vi "Handle Command.vi"(8 "error in (no error)":errorcluster, 9 "Data":variant, 10 "Command":string, 11 "Instrument.Oxford1820 in":refnum<class "Instrument.Oxford1820.lvclass">) -> (0 "error out":errorcluster, 1 "Processed Data":variant, 2 "Command":string, 3 "Instrument.Oxford1820 out":refnum<class "Instrument.Oxford1820.lvclass">)   [LabVIEW 2016, in "Instrument.Oxford1820.lvclass"]
uses:
  Instrument.Oxford1820.lvclass
  Typedefs/Instrument.Oxford1820.Commands-enum.ctl
  <instrlib>/Mercury iXX/Public/Libraries/Magnet/Controls/PSU Actions.ctl
  Typedefs/Targets.ctl
  Typedefs/PrivateEvents--Instrument.Oxford1820.SequenceSetMagnetField.ctl
  Typedefs/Instrument.Oxford1820.setMagnet-cluster.ctl
  <userlib>/LevyLab/Levylab Instruments/Instrument Types/Cryostat/Instrument.Cryostat.lvclass
  <instrlib>/Mercury iXX/Public/Libraries/Magnet.lvlib
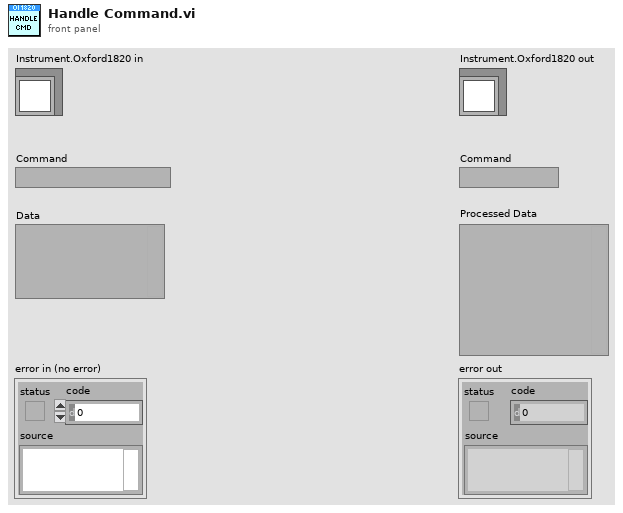
[diagram p1: front panel]
types:
  T1 = typedef "Instrument.Oxford1820.lvclass/Instrument.Oxford1820.Commands-enum.ctl" = enum16{"setAction", "setTarget", "setSwitchHeat", "setLambda", "setFillMode", "setNeedleValve", "setMagnetField", "getStatus", "getTarget", "getSwitchHeat", "getPSUField", "newcommand", "getMagnetField"}
  T2 = typedef "Mercury iXX.lvlib/Magnet.lvlib/PSU Actions.ctl" = string
  T3 = typedef "Instrument.Oxford1820.lvclass/Targets.ctl" = cluster{"Field (T)":dbl, "Field Rate (T/min)":dbl}
  T4 = typedef "Instrument.Oxford1820.lvclass/Instrument.Oxford1820.setMagnet-cluster.ctl" = cluster{"Target":T3, "persistent mode":bool}
  T5 = typedef "Instrument.Oxford1820.lvclass/PrivateEvents--Instrument.Oxford1820.SequenceSetMagnetField.ctl" = cluster{"setMagnet":T4}
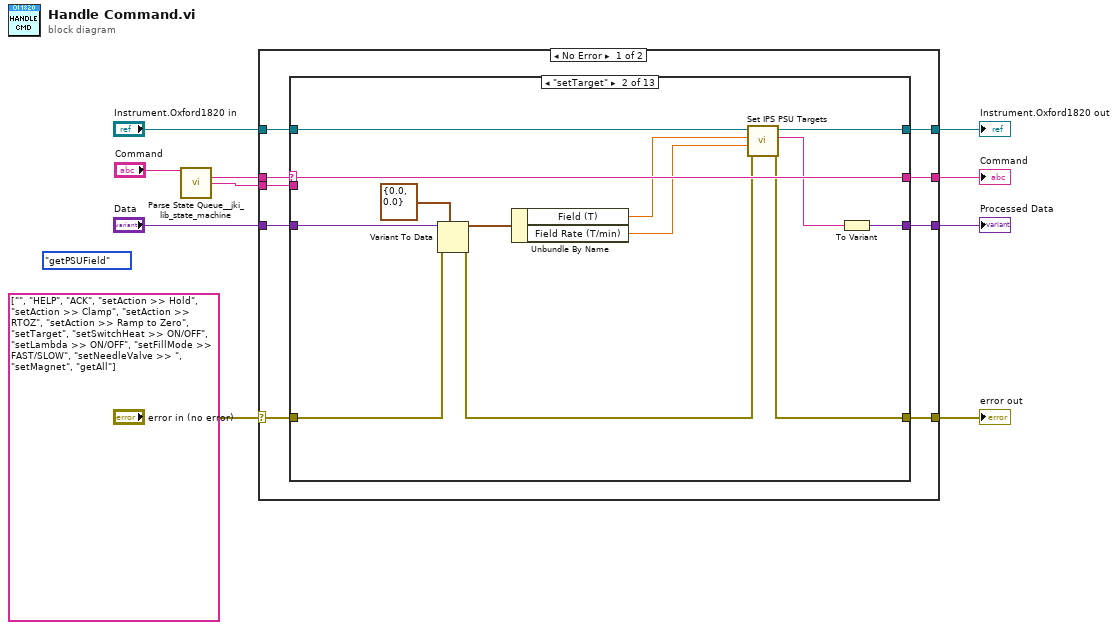
[diagram p0: block diagram]
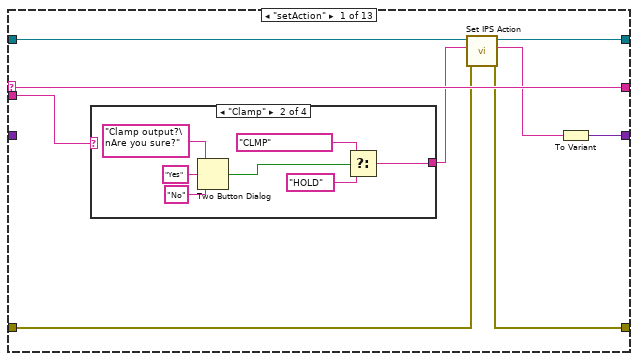
[diagram p2: hidden frame]
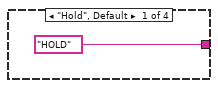
[diagram p3: hidden frame]
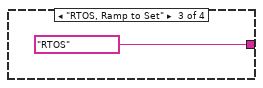
[diagram p4: hidden frame]
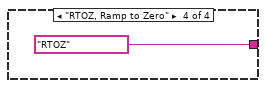
[diagram p5: hidden frame]
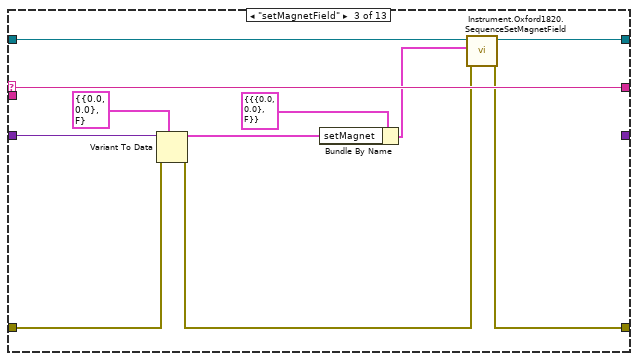
[diagram p6: hidden frame]
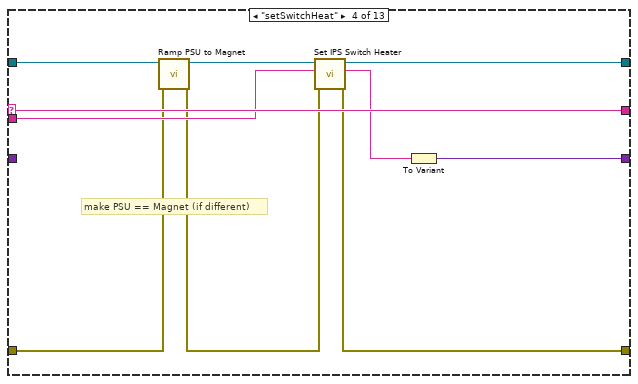
[diagram p7: hidden frame]
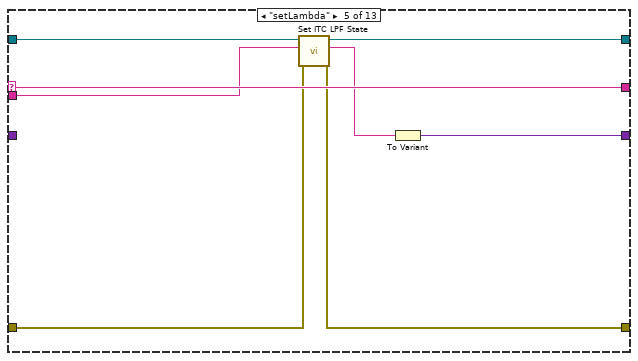
[diagram p8: hidden frame]
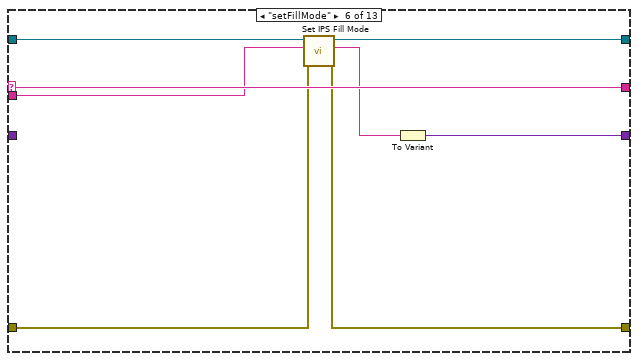
[diagram p9: hidden frame]
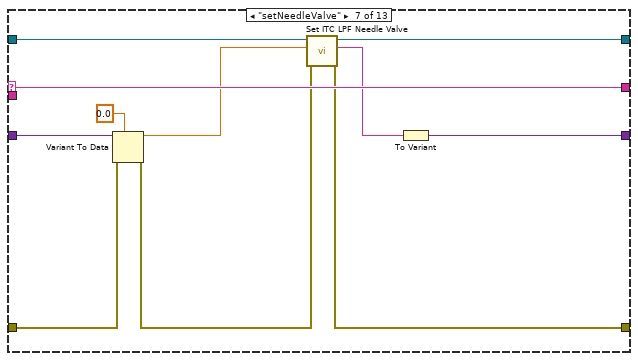
[diagram p10: hidden frame]
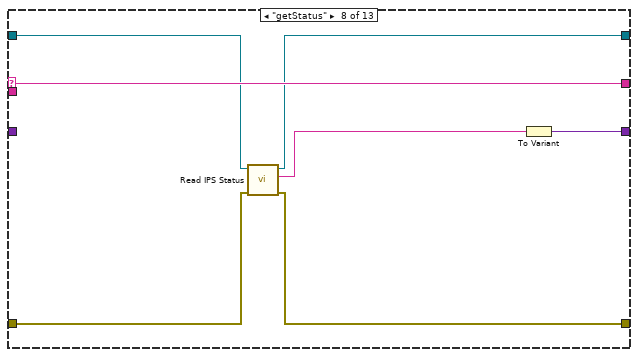
[diagram p11: hidden frame]
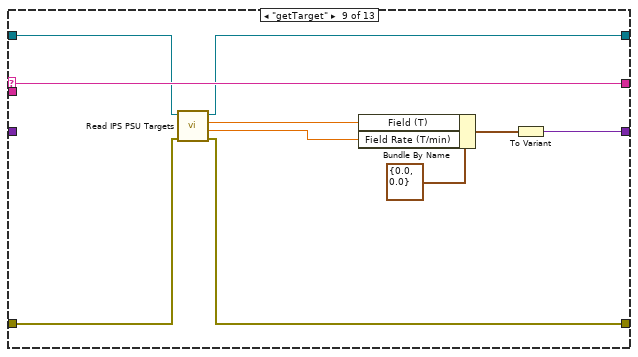
[diagram p12: hidden frame]
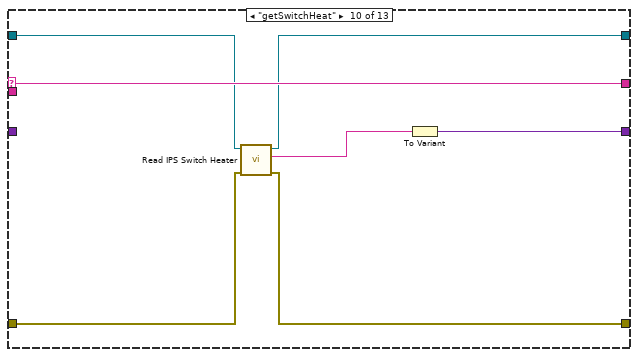
[diagram p13: hidden frame]
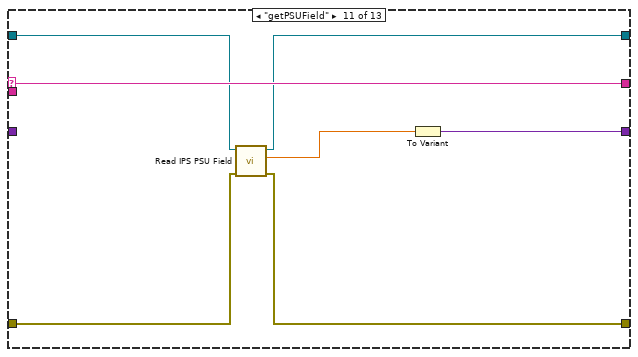
[diagram p14: hidden frame]
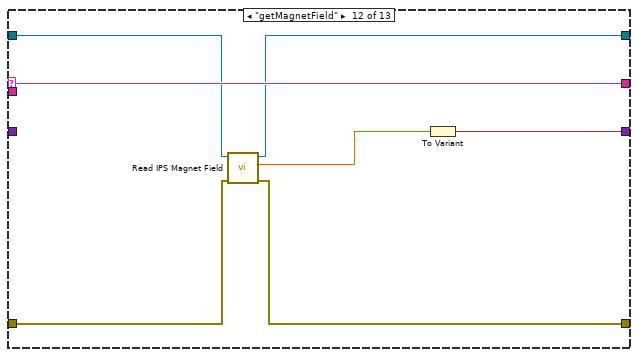
[diagram p15: hidden frame]
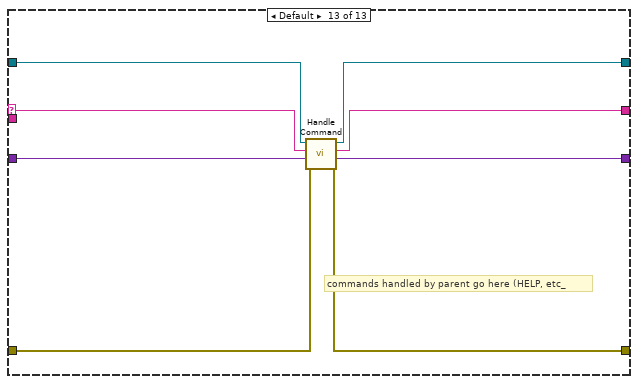
[diagram p16: hidden frame]
diagram:
  (unwired) Instrument.Oxford1820.Commands-enum."getPSUField" ("Commands")
  (unwired) string[] ["", "HELP", "ACK", "setAction >> Hold", "setAction >> Clamp", "setAction >> RTOZ", "setAction >> Ramp to Zero", "setTarget", "setSwitchHeat >> ON/OFF", "setLambda >> ON/OFF", "setFillMode >> FAST/SLOW", "setNeedleValve >> ", "setMagnet", "getAll"] ("Commands")
  n1 = call <vilib>:"Parse State Queue__jki_lib_state_machine.vi"("State Queue"="Command") -> ("Current State"=w2:string, "Arguments"=w1:string)  [unwired: 12 in, 1 out]
  n2 = case shown="No Error" "error in (no error)" {
    selector: "error in (no error)" -> [w14 w146]
    tunnel: [w13 w146] -> w10
    tunnel: [w19 _] -> w9
    tunnel: [w18 _] -> w8
    tunnel: [w17 w147] -> w7
    tunnel: "Data" -> [w16 _]
    tunnel: w2 -> [w11 _]
    tunnel: "Instrument.Oxford1820 in" -> [w15 w147]
    tunnel: w1 -> [w12 _]
    frame No Error {
      n3 = case shown="\"setTarget\"" w11 {
        selector: w11 -> [w28 w51 w62 w72 w80 w88 w99 w106 w116 w123 w130 w137 w138]
        tunnel: [w20 w46 _ w68 w75 w83 w94 w105 w115 w122 w129 w136 w145] -> w19
        tunnel: [w28 w51 w62 w72 w80 w88 w99 w106 w116 w123 w130 w137 w144] -> w18
        tunnel: [w25 w49 w60 w71 w78 w86 w97 w100 w108 w120 w127 w135 w143] -> w17
        tunnel: w16 -> [_ w45 w58 _ _ _ w92 _ _ _ _ _ w142]
        tunnel: w15 -> [w26 w50 w61 w66 w79 w87 w98 w101 w107 w121 w128 w131 w141]
        tunnel: w14 -> [w24 w40 w57 w64 w74 w82 w90 w104 w110 w119 w126 w133 w140]
        tunnel: [w23 w48 w59 w70 w77 w85 w96 w103 w109 w118 w125 w132 w139] -> w13
        tunnel: w12 -> [w27 _ _ w67 w73 w81 _ _ _ _ _ _ _]
        frame "setAction" {
          n4 = case shown="\"Clamp\"" w27 {
            tunnel: [T2 "HOLD" ("PSU Act Stat") w35 T2 "RTOS" ("PSU Act Stat") T2 "RTOZ" ("PSU Act Stat")] -> w22
            frame "Hold", Default {
            }
            frame "Clamp" {
              n5 = Two Button Dialog(message="Clamp output?\nAre you sure?", 1:"No" ("F button name (\"Cancel\")"), 2:"Yes" ("T button name (\"OK\")")) -> (T button?=w34:bool)
              n6 = Select(t=T2 "CLMP" ("PSU Act Stat"), s=w34, f=T2 "HOLD" ("PSU Act Stat")) -> (s? t:f=w35:T2)
            }
            frame "RTOS, Ramp to Set" {
            }
            frame "RTOZ, Ramp to Zero" {
            }
          }
          n7 = call "Set IPS Action.vi"("error in (no error)"=w24, "PSU Act Stat"=w22, "Instrument.Oxford1820 in"=w26) -> ("error out"=w23:errorcluster, "Response"=w21:string, "Instrument.Oxford1820 out"=w25:refnum<class "Instrument.Oxford1820.lvclass">)  [unwired: 6 in]
          n8 = To Variant(anything=w21) -> (Variant=w20:variant)
        }
        frame "setTarget" {
          n9 = Variant To Data(error in=w40, type=T3 {"Field (T)"=0.0, "Field Rate (T/min)"=0.0} ("Targets"), Variant=w45) -> (data=w43:T3, error out=w39:errorcluster)
          n10 = Unbundle By Name(w43) -> ("Field (T)"=w42:dbl, "Field Rate (T/min)"=w41:dbl)
          n11 = call "Set IPS PSU Targets.vi"("error in (no error)"=w39, "Target Field Rate (T/min)"=w41, "Target Field (T)"=w42, "Instrument.Oxford1820 in"=w50) -> ("error out"=w48:errorcluster, "Response"=w47:string, "Instrument.Oxford1820 out"=w49:refnum<class "Instrument.Oxford1820.lvclass">)  [unwired: 5 in]
          n12 = To Variant(anything=w47) -> (Variant=w46:variant)
        }
        frame "setMagnetField" {
          n13 = Variant To Data(error in=w57, type=T4 {"Target"={"Field (T)"=0.0, "Field Rate (T/min)"=0.0}, "persistent mode"=FALSE} ("output cluster"), Variant=w58) -> (data=w52:T4, error out=w56:errorcluster)
          n14 = Bundle By Name(cluster=T5 {"setMagnet"={"Target"={"Field (T)"=0.0, "Field Rate (T/min)"=0.0}, "persistent mode"=FALSE}} ("Set Magnet Field"), "setMagnet"=w52) -> (w54:T5)
          n15 = call "Instrument.Oxford1820.SequenceSetMagnetField.vi"("error in (no error)"=w56, "Set Magnet Field"=w54, "Instrument.Oxford1820"=w61) -> ("error out"=w59:errorcluster, "Instrument.Oxford1820 out"=w60:refnum<class "Instrument.Oxford1820.lvclass">)  [unwired: 7 in]
        }
        frame "setSwitchHeat" {
          # "make PSU == Magnet (if different)"
          n16 = call "Ramp PSU to Magnet.vi"("error in (no error)"=w64, "Instrument.Oxford1820 in"=w66) -> ("error out"=w63:errorcluster, "Instrument.Oxford1820 out"=w65:refnum<class "Instrument.Oxford1820.lvclass">)  [unwired: 8 in]
          n17 = call "Set IPS Switch Heater.vi"("error in (no error)"=w63, "Switch Heater Status"=w67, "Instrument.Oxford1820 in"=w65) -> ("error out"=w70:errorcluster, "Response"=w69:string, "Instrument.Oxford1820 out"=w71:refnum<class "Instrument.Oxford1820.lvclass">)  [unwired: 6 in]
          n18 = To Variant(anything=w69) -> (Variant=w68:variant)
        }
        frame "setLambda" {
          n19 = call "Set ITC LPF State.vi"("error in (no error)"=w74, "LPF State"=w73, "Instrument.Oxford1820 in"=w79) -> ("error out"=w77:errorcluster, "Response"=w76:string, "Instrument.Oxford1820 out"=w78:refnum<class "Instrument.Oxford1820.lvclass">)  [unwired: 6 in]
          n20 = To Variant(anything=w76) -> (Variant=w75:variant)
        }
        frame "setFillMode" {
          n21 = call "Set IPS Fill Mode.vi"("error in (no error)"=w82, "Fill Mode"=w81, "Instrument.Oxford1820 in"=w87) -> ("error out"=w85:errorcluster, "Response"=w84:string, "Instrument.Oxford1820 out"=w86:refnum<class "Instrument.Oxford1820.lvclass">)  [unwired: 6 in]
          n22 = To Variant(anything=w84) -> (Variant=w83:variant)
        }
        frame "setNeedleValve" {
          n23 = Variant To Data(error in=w90, type=0.0 ("Percentage Open (%)"), Variant=w92) -> (data=w91:dbl, error out=w89:errorcluster)
          n24 = call "Set ITC LPF Needle Valve.vi"("error in (no error)"=w89, "Percentage Open (%)"=w91, "Instrument.Oxford1820 in"=w98) -> ("error out"=w96:errorcluster, "Response"=w95:string, "Instrument.Oxford1820 out"=w97:refnum<class "Instrument.Oxford1820.lvclass">)  [unwired: 6 in]
          n25 = To Variant(anything=w95) -> (Variant=w94:variant)
        }
        frame "getStatus" {
          n26 = call "Read IPS Status.vi"("error in (no error)"=w104, "Instrument.Oxford1820 in"=w101) -> ("error out"=w103:errorcluster, "Status"=w102:string, "Instrument.Oxford1820 out"=w100:refnum<class "Instrument.Oxford1820.lvclass">)  [unwired: 7 in]
          n27 = To Variant(anything=w102) -> (Variant=w105:variant)
        }
        frame "getTarget" {
          n28 = call "Read IPS PSU Targets.vi"("error in (no error)"=w110, "Instrument.Oxford1820 in"=w107) -> ("error out"=w109:errorcluster, "Target Field Rate (T/min)"=w111:dbl, "Target Field (T)"=w112:dbl, "Instrument.Oxford1820 out"=w108:refnum<class "Instrument.Oxford1820.lvclass">)  [unwired: 6 in]
          n29 = Bundle By Name(cluster=T3 {"Field (T)"=0.0, "Field Rate (T/min)"=0.0} ("Target"), "Field (T)"=w112, "Field Rate (T/min)"=w111) -> (w114:T3)
          n30 = To Variant(anything=w114) -> (Variant=w115:variant)
        }
        frame "getSwitchHeat" {
          n31 = call "Read IPS Switch Heater.vi"("error in (no error)"=w119, "Instrument.Oxford1820 in"=w121) -> ("error out"=w118:errorcluster, "Switch Heater Status"=w117:string, "Instrument.Oxford1820 out"=w120:refnum<class "Instrument.Oxford1820.lvclass">)  [unwired: 6 in, 1 out]
          n32 = To Variant(anything=w117) -> (Variant=w122:variant)
        }
        frame "getPSUField" {
          n33 = call "Read IPS PSU Field.vi"("error in (no error)"=w126, "Instrument.Oxford1820 in"=w128) -> ("error out"=w125:errorcluster, "Power Supply Field (T)"=w124:dbl, "Instrument.Oxford1820 out"=w127:refnum<class "Instrument.Oxford1820.lvclass">)  [unwired: 7 in]
          n34 = To Variant(anything=w124) -> (Variant=w129:variant)
        }
        frame "getMagnetField" {
          n35 = call "Read IPS Magnet Field.vi"("error in (no error)"=w133, "Instrument.Oxford1820 in"=w131) -> ("error out"=w132:errorcluster, "Magnet Field (T)"=w134:dbl, "Instrument.Oxford1820 out"=w135:refnum<class "Instrument.Oxford1820.lvclass">)  [unwired: 7 in]
          n36 = To Variant(anything=w134) -> (Variant=w136:variant)
        }
        frame Default {
          # "commands handled by parent go here (HELP, etc_"
          n37 = call-parent "Handle Command.vi"("error in (no error)"=w140, "Data"=w142, "Command"=w138, "Instrument in"=w141) -> ("error out"=w139:errorcluster, "Processed Data"=w145:variant, "Command"=w144:string, "Instrument out"=w143:refnum<class "Instrument.Oxford1820.lvclass">)  [unwired: 4 in]
        }
      }
    }
    frame Error {
    }
  }
  "error out" <- w10
  "Instrument.Oxford1820 out" <- w7
  "Processed Data" <- w9
  "Command" <- w8
